vi "LoadSystemDefinition.vi"(8 "error in (no error)":errorcluster, 11 "SysDef.Path":path) -> (0 "error out":errorcluster, 2 "Aliases.Outputs":T1[](array[typedef]), 3 "Aliases.All":T1[](array[typedef]))   [LabVIEW 2013]
uses:
  Types/ChannelProperties.ctl
  NationalInstruments.VeriStand.SystemStorage
  NationalInstruments.VeriStand.SystemDefinitionAPI
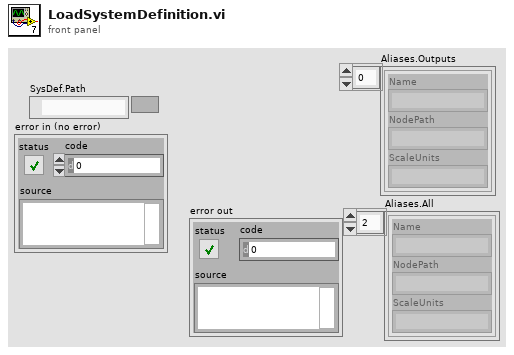
[diagram p1: front panel]
types:
  T1 = typedef "ChannelProperties.ctl" = cluster{"Name":string, "NodePath":string, "ScaleUnits":string}
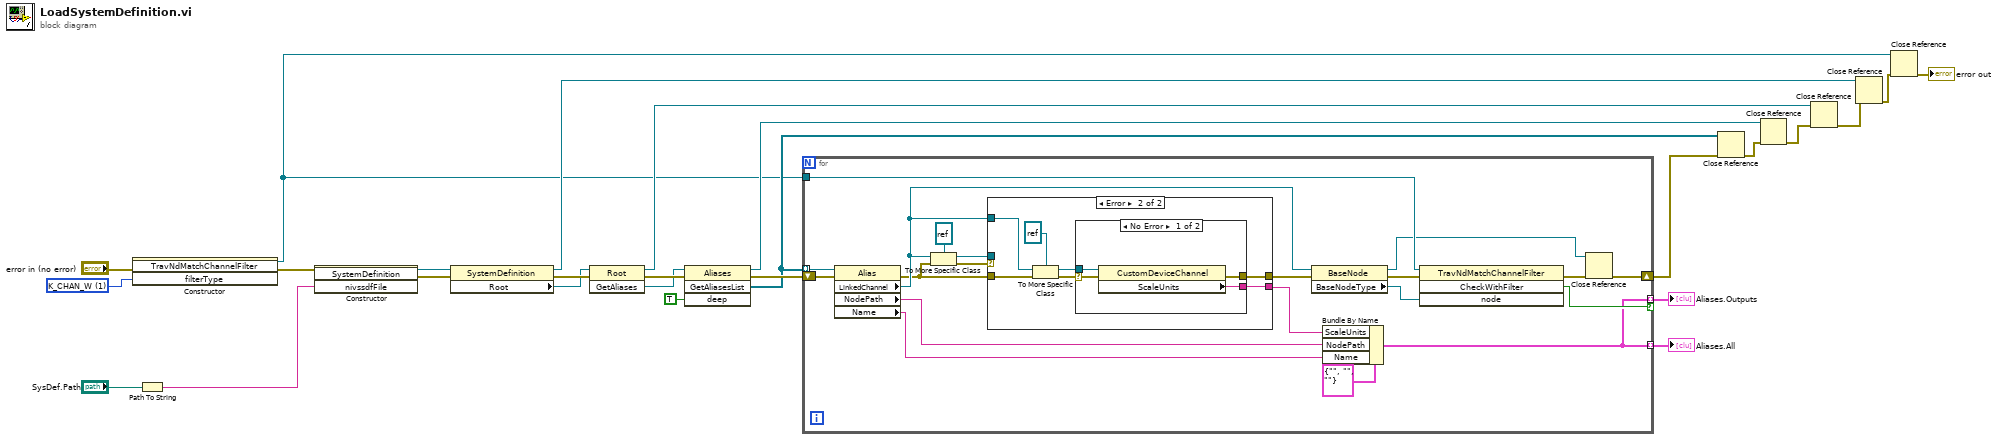
[diagram p0: block diagram]
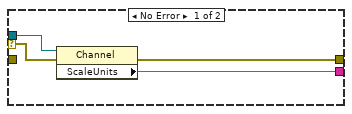
[diagram p2: hidden frame]
diagram:
  w16 = u8 1 items=["K_CHAN_R", "K_CHAN_W", "K_CHAN_VOLT", "K_CHAN_FAULT"] ("filterType")
  n1 = constructor class="TravNdMatchChannelFilter"(error in="error in (no error)", "filterType"=w16) -> (reference out=w9:refnum<k24>, error out=w14:errorcluster)  [unwired: 2 in, 2 out]
  n2 = Path To String(path="SysDef.Path") -> (string=w19:string)
  n3 = constructor class="SystemDefinition"(error in=w14, "nivssdfFile"=w19) -> (reference out=w20:refnum<k24>, error out=w25:errorcluster)  [unwired: 2 in, 2 out]
  n4 = property class="SystemDefinition"(reference=w20, error in=w25) -> (reference out=w13:refnum<k24>, error out=w24:errorcluster, "Root"=w21:refnum<k24>)
  n5 = invoke class="Root" method="GetAliases"(reference=w21, error in=w24) -> (reference out=w12:refnum<k24>, error out=w23:errorcluster, "GetAliases"=w17:refnum<k24>)  [unwired: 1 in]
  n6 = invoke class="Aliases" method="GetAliasesList"(reference=w17, error in=w23, "deep"=TRUE) -> (reference out=w11:refnum<k24>, error out=w26:errorcluster, "GetAliasesList"=w10:refnum<k24>[])  [unwired: 1 in, 1 out]
  n7 = for {
    tunnel: w10 -> [w46] mode=indexing
    tunnel: [w27] -> w2 mode=indexing if=w44
    shift-right: [w40] -> w4
    shift-left: w26 -> [w45]
    tunnel: [w27] -> w1 mode=indexing
    tunnel: w9 -> [w42]
    n8 = property class="Alias"(reference=w46, error in=w45) -> (error out=w35:errorcluster, "LinkedChannel"=w36:refnum<k24>, "NodePath"=w29:string, "Name"=w31:string)  [unwired: 1 out]
    n9 = To More Specific Class(target class=refnum<k24> refnum ("new reference"), reference=w36, error in=w35) -> (specific class reference=w38:refnum<k24>, error out=w39:errorcluster)
    n10 = case shown="Error" w39 {
      selector: w39 -> [w49 _]
      tunnel: w38 -> [w50 _]
      tunnel: [w47 w52] -> w34
      tunnel: w36 -> [_ w57]
      tunnel: w35 -> [_ w56]
      tunnel: [w48 w51] -> w28
      frame No Error {
        n11 = property class="Channel"(reference=w50, error in=w49) -> (error out=w47:errorcluster, "ScaleUnits"=w48:string)  [unwired: 1 out]
      }
      frame Error {
        n12 = To More Specific Class(target class=refnum<k24> refnum ("new reference"), reference=w57, error in=w56) -> (specific class reference=w54:refnum<k24>, error out=w53:errorcluster)
        n13 = case shown="No Error" w53 {
          selector: w53 -> [w60 _]
          tunnel: w54 -> [w61 _]
          tunnel: [w59 _] -> w52
          tunnel: [w58 _] -> w51
          frame No Error {
            n14 = property class="CustomDeviceChannel"(reference=w61, error in=w60) -> (error out=w59:errorcluster, "ScaleUnits"=w58:string)  [unwired: 1 out]
          }
          frame Error {
          }
        }
      }
    }
    n15 = property class="BaseNode"(reference=w36, error in=w34) -> (reference out=w33:refnum<k24>, error out=w43:errorcluster, "BaseNodeType"=w41:refnum<k24>)
    n16 = Bundle By Name(cluster=T1 {"Name"="", "NodePath"="", "ScaleUnits"=""}, "ScaleUnits"=w28, "NodePath"=w29, "Name"=w31) -> (w27:T1)
    n17 = invoke class="TravNdMatchChannelFilter" method="CheckWithFilter"(reference=w42, error in=w43, "node"=w41) -> (error out=w32:errorcluster, "CheckWithFilter"=w44:bool)  [unwired: 1 in, 2 out]
    n18 = Close Reference(reference=w33, error in (no error)=w32) -> (error out=w40:errorcluster)
  }
  "Aliases.Outputs" <- w2
  "Aliases.All" <- w1
  n19 = Close Reference(reference=w10, error in (no error)=w4) -> (error out=w8:errorcluster)
  n20 = Close Reference(reference=w11, error in (no error)=w8) -> (error out=w7:errorcluster)
  n21 = Close Reference(reference=w12, error in (no error)=w7) -> (error out=w6:errorcluster)
  n22 = Close Reference(reference=w13, error in (no error)=w6) -> (error out=w5:errorcluster)
  n23 = Close Reference(reference=w9, error in (no error)=w5) -> (error out=→"error out":errorcluster)
